vi "SVT Exp Avg Sound Level.vi"   [LabVIEW 2017]
doc: "Computes the exponential averaged sound level of <B>scaled signal [EU]</B> based on <B>exponential mode</B> and returns the sound level for the signal in <B>exp avg sound level [dB EU]</B>. The SVT Exp Avg Sound Level VI returns the exponential average sound level computed after each individual sample of the time record. You can use this polymorphic VI to compute the exponential averaged sound level for a single channel or for N channels. The data type you wire to the <B>scaled signal [EU]</B> input determines the polymorphic instance to use."
uses:
  <vilib>/addons/Sound and Vibration/svt_Level/SoundVib_SoundLevel.lvlib
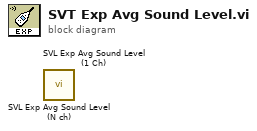
[diagram p0: block diagram]
diagram:
  n1 = call <vilib>:"SVL Exp Avg Sound Level (N ch).vi"() -> ()  [unwired: 7 in, 5 out]
  n2 = call <vilib>:"SVL Exp Avg Sound Level (1 Ch).vi"() -> ()  [unwired: 7 in, 5 out]
